vi "Load_from_Project.vi"(8 "error in (no error)":errorcluster, 9 "index":string, 10 "buildObject":T1, 11 "IB_RegDest in":refnum<class "IB_RegDest.lvclass">) -> (0 "error out":errorcluster, 1 "index out":string, 2 "buildObject out":T1, 3 "IB_RegDest out":refnum<class "IB_RegDest.lvclass">)   [LabVIEW 2020, in "IB_RegDest.lvclass"]
uses:
  <vilib>/AppBuilder/IB_Classes/RegDest/IB_RegDest.lvclass
  <vilib>/AppBuilder/IB_Classes/RegDest/IB_RegDest.lvclass/IB_RegDest.ctl
  <vilib>/AppBuilder/IB_RW_Project/IB_RW_Project_PropBag_Action.ctl
  <resource>/Framework/Providers/API/ItemRef.ctl
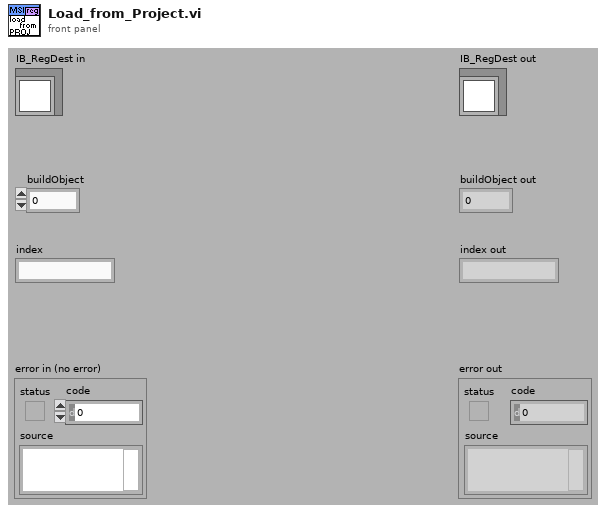
[diagram p1: front panel]
types:
  T1 = typedef "ItemRef.ctl" = u64
  T2 = typedef "IB_RW_Project_PropBag_Action.ctl" = enum16{"read", "write", "clear", "readPrevious", "writePrevious", "clearPrevious"}
  T3 = typedef "IB_RW_Project_RegDest_Data.ctl" = cluster{"parentTag":string, "dirTag":string, "dirName":string, "unlock":bool}
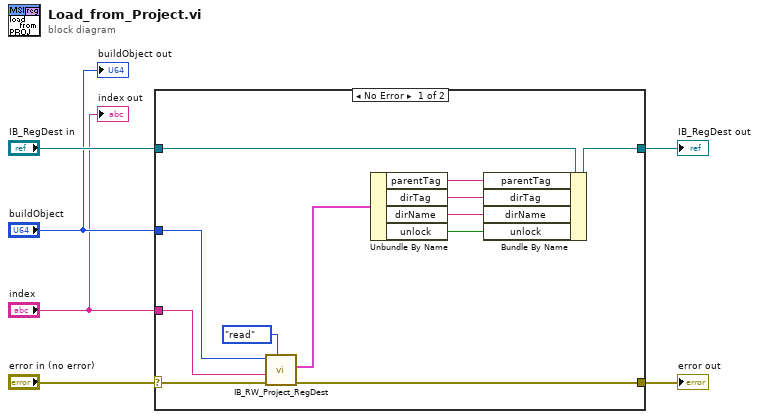
[diagram p0: block diagram]
diagram:
  n1 = case shown="No Error" "error in (no error)" {
    selector: "error in (no error)" -> [w8 w20]
    tunnel: [w7 w20] -> w5
    tunnel: [w13 w19] -> w3
    tunnel: "IB_RegDest in" -> [w14 w19]
    tunnel: "buildObject" -> [w17 _]
    tunnel: "index" -> [w18 _]
    frame No Error {
      n2 = call <vilib>:"IB_RW_Project_RegDest.vi"("action"=IB_RW_Project_PropBag_Action."read", "error in (no error)"=w8, "index in"=w18, "buildObject"=w17) -> ("error out"=w7:errorcluster, "RegDest"=w15:T3)  [unwired: 1 in, 5 out]
      n3 = Unbundle By Name(w15) -> ("parentTag"=w12:string, "dirTag"=w11:string, "dirName"=w10:string, "unlock"=w9:bool)
      n4 = Bundle By Name(cluster=w14, "parentTag"=w12, "dirTag"=w11, "dirName"=w10, "unlock"=w9) -> (w13:refnum<class "IB_RegDest.lvclass">)
    }
    frame Error {
    }
  }
  "error out" <- w5
  "IB_RegDest out" <- w3
  "buildObject out" <- "buildObject"
  "index out" <- "index"
